vi "LED_Metronome.vi"() -> ()   [LabVIEW 2022 SP3]
panel:
  in  "BPM":i64
  in  "?":bool
  out "LED":bool
  # "LED_Metronome:\nEnter an integar value for BPM\nto see the LED blink that many times\nin a minute."
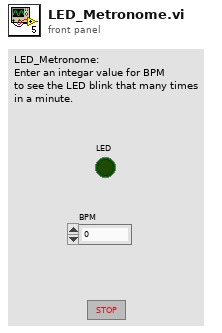
[diagram p1: front panel]
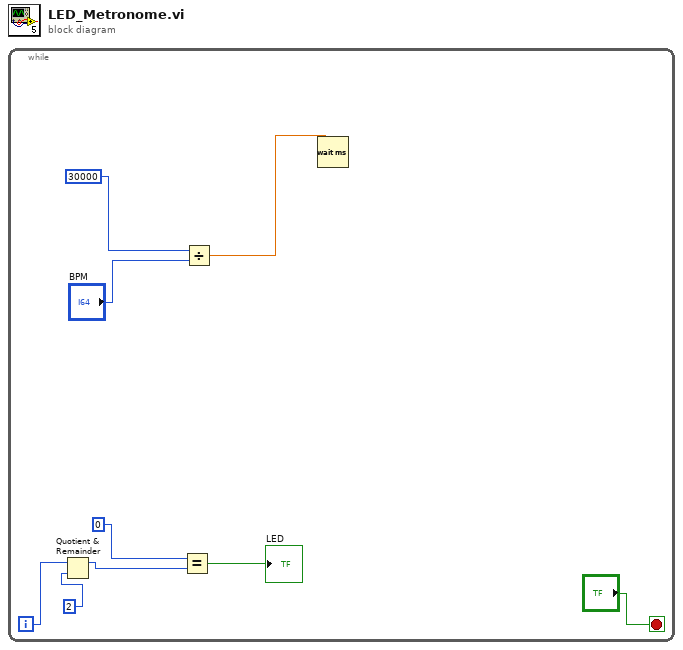
[diagram p0: block diagram]
diagram:
  n1 = while {
    i -> [w6]
    stop <- "?" stop-if-true
    n2 = Quotient & Remainder(x=w6, y=2) -> (x-y*floor(x/y)=w3:i32)  [unwired: 1 out]
    n3 = Equal?(x=0, y=w3) -> (x = y?=→"LED":bool)
    n4 = Divide(x=30000, y="BPM") -> (x/y=w7:dbl)
    n5 = Wait (ms)(milliseconds to wait=w7) -> ()  [unwired: 1 out]
  }
